vi "Nanotec Controller.vi"(6 "remote":T1) -> ()   [LabVIEW 2023, in "Nanotec Controller.lvlib"]
uses:
  Nanotec Controller.lvlib
  controls/Drive-Mode.ctl
  controls/Go.ctl
  controls/Velocity Pams.ctl
  controls/Units.ctl
  controls/Exps.ctl
  controls/Times.ctl
  controls/Profile Position Units.ctl
  <extravilib>/ChannelInstances/Messenger-t'Message Queue.lvlib-Message Cluster.ctl'/))Channel.ctl
  CMH-Lib/Message Queue/Message Cluster.ctl
  CMH-Lib/Message Queue/Enqueue Multiple Messages.vi
  <extravilib>/ChannelInstances/Messenger-t'Message Queue.lvlib-Message Cluster.ctl'/Read.vi
  <extravilib>/ChannelInstances/Messenger-t'Message Queue.lvlib-Message Cluster.ctl'/Write With Abort.vi
  <extravilib>/ChannelInstances/Messenger-t'Message Queue.lvlib-Message Cluster.ctl'/Read With Abort.vi
  <extravilib>/ChannelInstances/Event Messenger-bool/Instantiate.vi
  <extravilib>/ChannelInstances/Event Messenger-bool/))Channel.vi
  <extravilib>/ChannelInstances/Messenger-t'Message Queue.lvlib-Message Cluster.ctl'/Endpoint.vi
  <vilib>/Utility/error.llb/Error Cluster From Error Code.vi
  <vilib>/ErrorRing/Error Ring.xnode
  CMH-Lib/Message Queue.lvlib
  <extravilib>/ChannelInstances/Event Messenger-bool.lvlib
  NanoLibDLL.dll
  CMH-Lib/Message Queue Helper.lvlib
  <extravilib>/ChannelInstances/Messenger-t'Message Queue.lvlib-Message Cluster.ctl'.lvlib
panel:
  out "Log":string
  out "error out":errorcluster
  in  "Connection Status Control":enum32{"Connection", "Status"}(tab)
  in  "Connect Button":bool
  in  "Ports":i32(listbox)
  in  "Devices":i32(listbox)
  in  "Reboot Device":bool
  out "Connected":bool
  out "NanoJ: STOPPED":bool
  out "Fault":bool
  out "Closed loop available":bool
  out "6041 Bit 13":bool
  out "Warning":bool
  out "Target reached":bool
  out "Internal limit reached":bool
  out "6041 Bit 12":bool
  out "Quick Stop":bool
  out "Voltage enabled":bool
  out "CiA 402 State":string
  out "Mode":string
  in  "Auto-refresh":bool
  out "Current Position":i32
  in  "Get Exceptions":bool
  in  "Get Error Stack":bool
  in  "Device Error Stack":i32(listbox)
  in  "Quick Stop":bool
  in  "Mode Control":T2(tab)
  in  "Open Loop Idle Current (mA)":u32
  in  "Set Motor Settings Button":bool
  in  "Save Motorpams Button":bool
  in  "Auto-Setup Motor Parameters":bool
  in  "Pole Pair Count":u32
  in  "Max Duration (ms)":u32
  in  "Max Current (mA)":u32
  in  "Rated Current (mA)":u32
  in  "Drive-Mode":T3=8 items=["BLDC"=65, "Stepper Closed Loop"=1, "Stepper Open Loop without current-reduction"=0, "Stepper Open Loop with current-reduction"=8]
  in  "Profile Position Units":T4 {"Positioning Exp" items=["10^6"=6, "10^5"=5, "10^4"=4, "10^3"=3, "10^2"=2, "10^1"=1, "10^0"=0, "10^-1"=255, "10^-2"=254, "10^-3"=253, "10^-4"=252, "10^-5"=251, "10^-6"=250]; "Positioning Unit" items=["meter"=1, "inch"=193, "foot"=194, "grade"=64, "radian"=16, "degree"=65, "arcminute"=66, "arcsecond"=67, "mechanical rev"=180]}
  in  "Profile Velocity Units":T8 {"Velocity Time" items=["second"=3, "minute"=71, "hour"=72, "day"=73, "year"=74]; "Velocity Exp" items=["10^6"=6, "10^5"=5, "10^4"=4, "10^3"=3, "10^2"=2, "10^1"=1, "10^0"=0, "10^-1"=255, "10^-2"=254, "10^-3"=253, "10^-4"=252, "10^-5"=251, "10^-6"=250]; "Velocity Unit" items=["meter"=1, "inch"=193, "foot"=194, "grade"=64, "radian"=16, "degree"=65, "arcminute"=66, "arcsecond"=67, "mechanical rev"=180]}
  in  "Gear Ratio Shaft Revs":u32
  in  "Gear Ratio Motor Revs":u32
  in  "Shaft Revolutions":u32
  in  "Save User Units Button":bool
  in  "Set User Units Button":bool
  in  "Feed Constant Per":u32
  in  "Absolute/Relative":u32(ring) items=["Absolute", "Relative"]
  out "Set Position":i32
  in  "Profile Velocity":u32=1
  in  "Halt Positioning Button":bool
  in  "Start Positioning Button":T9
  in  "Target":i32(slide)
  in  "Save Velocity Pams":bool
  in  "Set Velocity Pams":bool
  in  "Velocity Pams":T10={"Target Velocity"=1, "Delta Speed Acc"=1, "Delta Time Acc"=1, "DeltaSpeed Dec"=1, "DeltaTime Dec"=1}
  out "Velocity Demanded":i16
  out "Velocity Actual":i16
  in  "Halt Velocity Button":bool
  in  "Start Velocity Button":T9
  in  "Homing Method":u32(ring)=17 items=["Referencing Negative Switch"=17]
  in  "Speed Switch":u32=3
  in  "Speed Zeroing":u32=2
  in  "Home Button":bool
  in  "Exceptions":i32(listbox)
  in  "Exit":bool
  # "ONLY NECESSARY AFTER\nMOTOR CHANGE"
  # "Position in User Units"
  # "1/min"
  # "<"
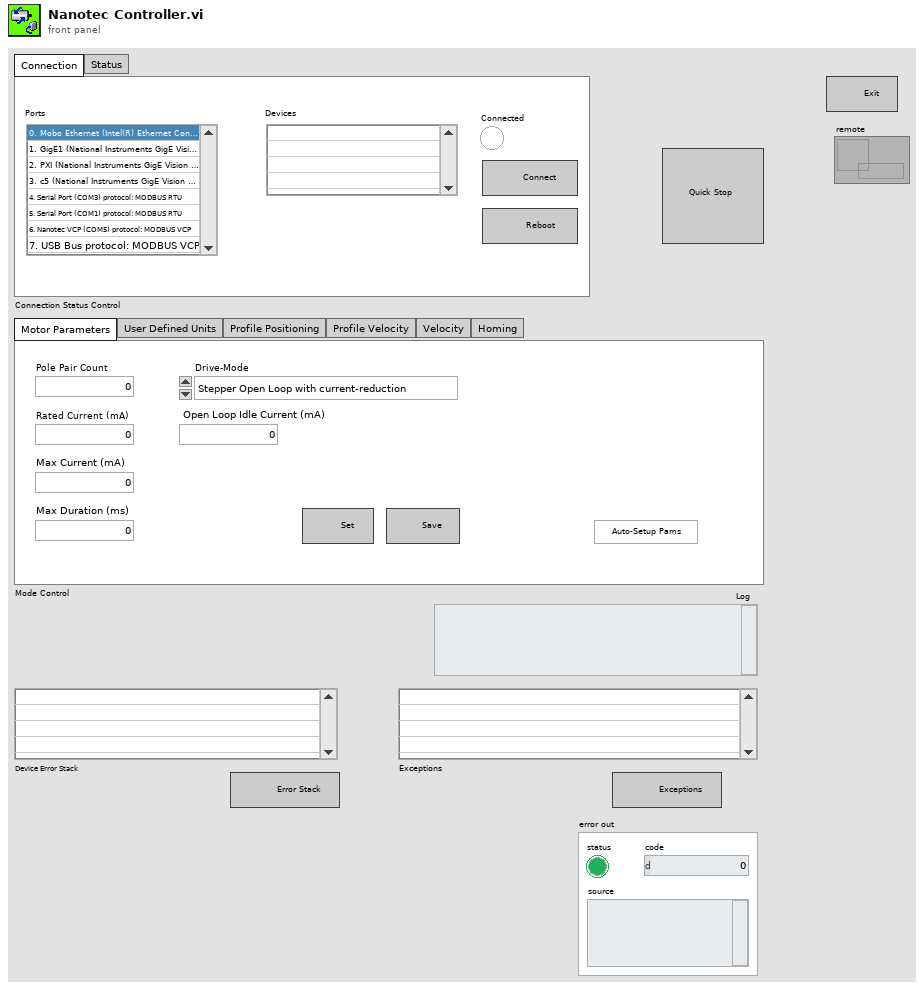
[diagram p1: front panel]
types:
  T1 = typedef "Messenger-t'Message Queue.lvlib-Message Cluster.ctl'.lvlib/))Channel.ctl" = refnum<queue>
  T2 = enum32{"Motor Parameters", "User Defined Units", "Profile Positioning", "Profile Velocity", "Velocity", "Homing"}
  T3 = typedef "Nanotec Controller.lvlib/Drive-Mode.ctl" = u32
  T4 = typedef "Nanotec Controller.lvlib/Profile Position Units.ctl" = cluster{"Positioning Unit":T5, "Positioning Exp":T6}
  T5 = typedef "Nanotec Controller.lvlib/Units.ctl" = u32
  T6 = typedef "Nanotec Controller.lvlib/Exps.ctl" = u32
  T7 = typedef "Nanotec Controller.lvlib/Times.ctl" = u32
  T8 = cluster{"Velocity Unit":T5, "Velocity Exp":T6, "Velocity Time":T7}
  T9 = typedef "Nanotec Controller.lvlib/Go.ctl" = bool
  T10 = typedef "Nanotec Controller.lvlib/Velocity Pams.ctl" = cluster{"Target Velocity":i16, "Delta Speed Acc":u32, "Delta Time Acc":u16, "DeltaSpeed Dec":u32, "DeltaTime Dec":u16}
  T11 = cluster{"Target Velocity":i16, "Delta Speed Acc":u32, "Delta Time Acc":u16, "DeltaSpeed Dec":u32, "DeltaTime Dec":u16}
  T12 = typedef "Event Messenger-bool.lvlib/))Channel.ctl" = refnum<queue>
  T13 = cluster{"velUnit":u32, "velExp":u32, "velTime":u32}
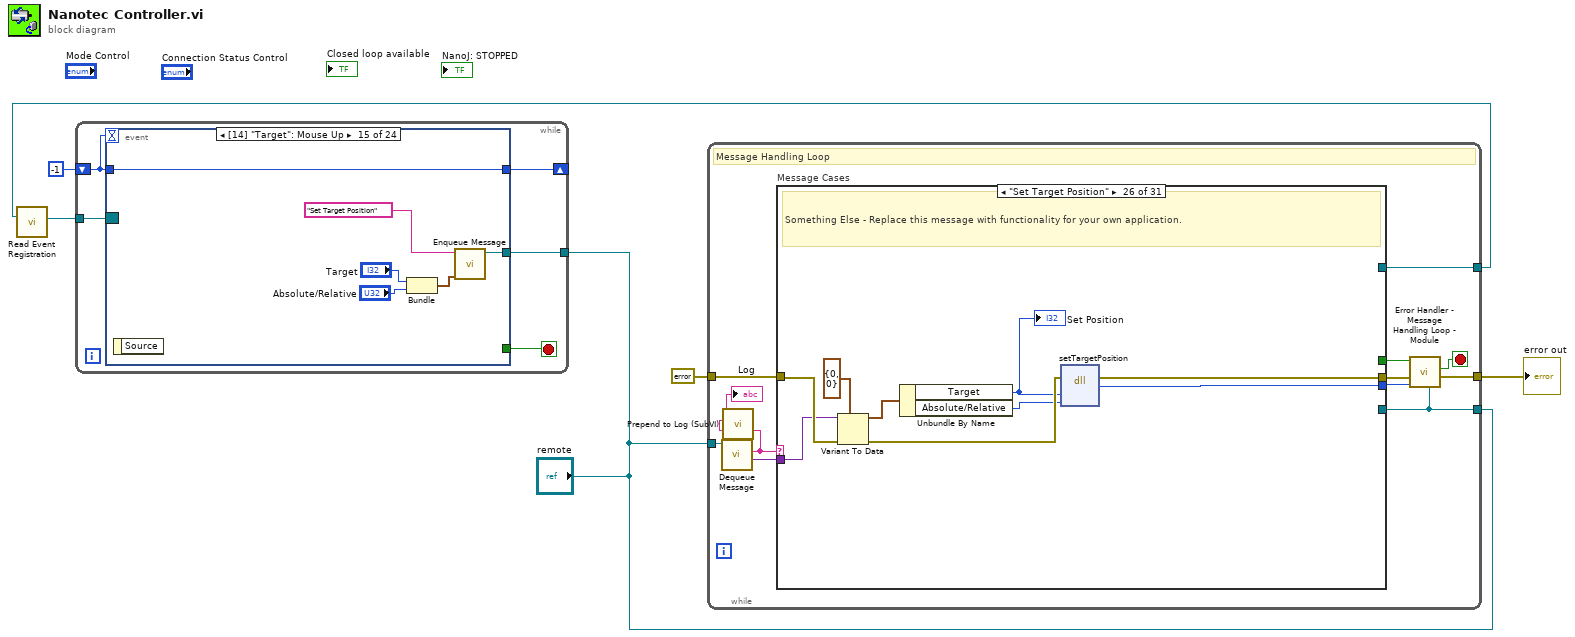
[diagram p0: block diagram]
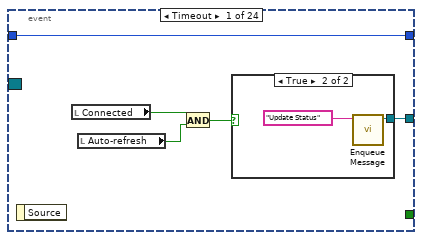
[diagram p2: hidden frame]
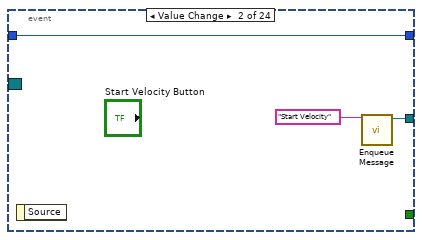
[diagram p4: hidden frame]
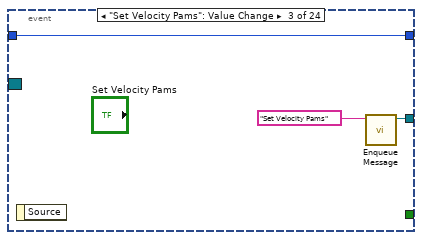
[diagram p5: hidden frame]
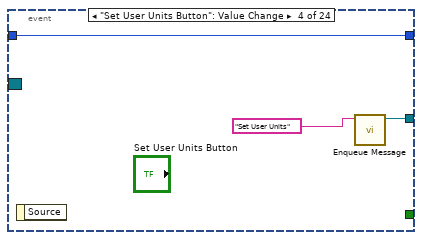
[diagram p6: hidden frame]
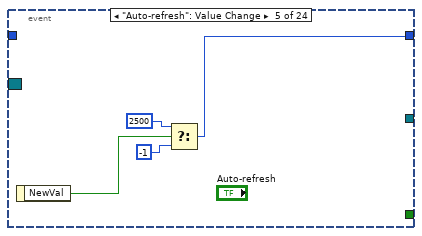
[diagram p7: hidden frame]
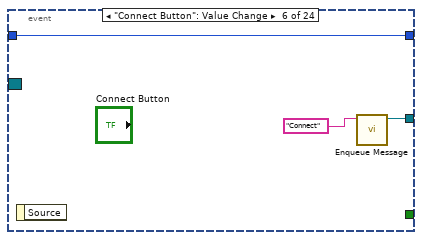
[diagram p8: hidden frame]
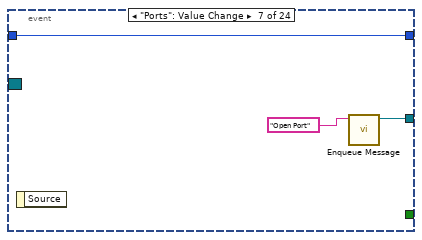
[diagram p9: hidden frame]
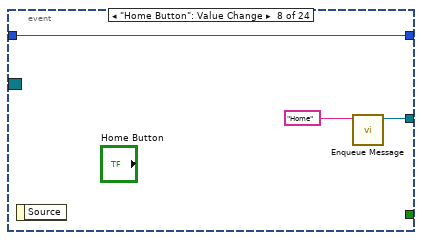
[diagram p10: hidden frame]
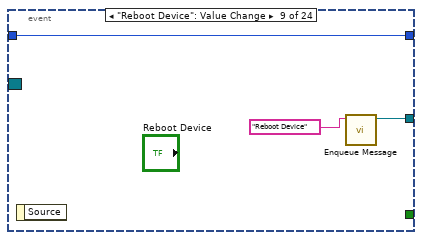
[diagram p11: hidden frame]
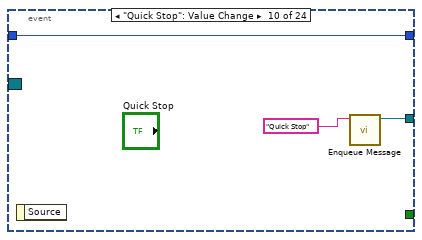
[diagram p12: hidden frame]
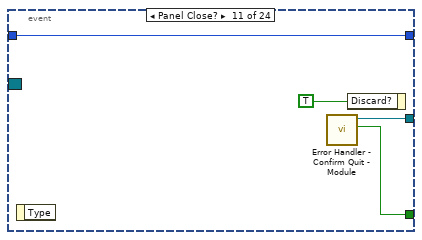
[diagram p13: hidden frame]
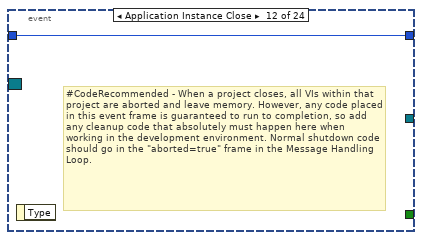
[diagram p14: hidden frame]
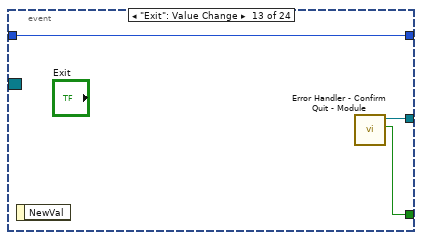
[diagram p15: hidden frame]
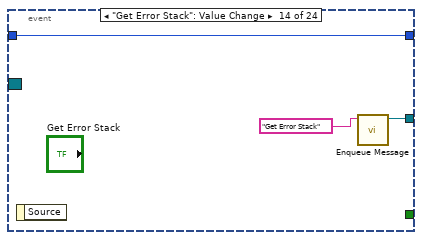
[diagram p16: hidden frame]
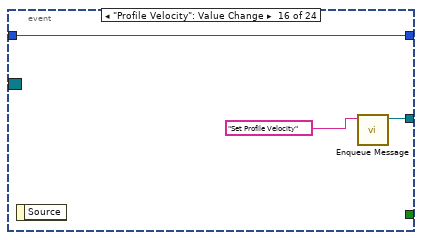
[diagram p17: hidden frame]
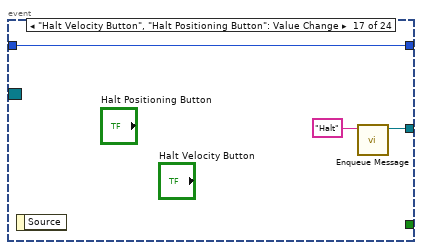
[diagram p18: hidden frame]
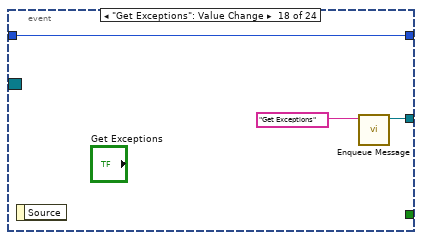
[diagram p19: hidden frame]
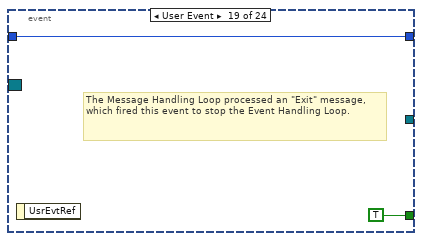
[diagram p20: hidden frame]
diagram:
  n1 = while {
    tunnel: [w15] -> w6
    tunnel: "remote" -> [w17]
    tunnel: errorcluster {"status"=FALSE, "code"=0, "source"=""} ("error IO") -> [w18]
    tunnel: "remote" -> [w7]
    tunnel: [w8] -> w2
    stop <- w12 stop-if-true
    # "Message Handling Loop"
    n2 = call "Dequeue Message.vi"("channel"=w17) -> ("message data"=w16:variant, "message"=w14:string)  [unwired: 8 in, 1 out]
    n3 = call "Prepend to Log (SubVI).vi"("new entry"=w14) -> ("Log out"=→"Log":string)  [unwired: 10 in]
    n4 = case "Message Cases" shown="\"Set Target Position\"" w14 {
      selector: w14 -> [_ _ _ _ _ _ _ _ _ _ _ _ _ _ _ _ _ _ _ _ _ _ _ _ _ _ _ _ _ _ w247]
      tunnel: w18 -> [w19 w27 w37 w46 w49 w55 w71 w74 w84 w91 w100 w105 w108 w129 w132 w136 w141 w153 w157 w161 w167 w170 w174 w189 w193 w200 w216 w219 w222 w243 _]
      tunnel: [w19 w21 w36 w45 w48 w54 w66 w73 w78 w85 w99 w104 w110 w128 w131 w137 w145 w151 w158 w162 w165 w169 w175 w188 w192 w202 w215 w218 w221 w225 w248] -> w10
      tunnel: w16 -> [_ w26 _ _ _ _ w70 _ _ _ _ _ _ _ _ _ _ _ _ _ _ _ _ _ _ w199 _ _ _ _ _]
      tunnel: [_ _ _ _ _ w50 w65 _ _ _ _ _ _ _ _ _ w147 w148 _ _ _ _ _ _ _ _ _ _ _ _ _] -> w7
      tunnel: [_ _ w35 w44 w47 w51 _ w72 _ _ w98 w103 w106 w127 w130 w135 _ w149 w156 w160 w166 w168 w171 w187 w191 w201 w214 w217 w220 w244 _] -> w11
      tunnel: [_ _ _ _ _ _ _ w76 _ _ _ _ _ _ _ _ _ _ _ _ _ _ _ _ _ _ _ _ _ _ _] -> w15
      tunnel: [_ _ _ _ _ _ _ TRUE _ _ _ _ _ _ _ _ FALSE _ _ _ _ _ _ _ _ _ _ _ _ _ _] -> w9
      frame "---Copy This Frame---" {
        # "Duplicate this frame when creating new messages.  Change this comment in the duplicated frame to describe this message."
      }
      frame "Log" {
        # "Duplicate this frame when creating new messages.  Change this comment in the duplicated frame to describe this message."
        n5 = Variant To Data(error in=w27, type="", Variant=w26) -> (data=w22:string, error out=w21:errorcluster)
        n6 = local read "Log"() -> (w24:string)
        n7 = Concatenate Strings(w22, "\r", w24) -> (w20:string)
        n8 = local write "Log"(w20) -> ()
      }
      frame "Get Velocity Pams" {
        # "Duplicate this frame when creating new messages.  Change this comment in the duplicated frame to describe this message."
        n9 = dll-call lib="NanoLibDLL.dll" fn="getVelocityPams"(error in=w37) -> (error out=w36:errorcluster, "success"=w35:i32, "targetVel"=w33:i16, "deltaSpeedAcc"=w32:u32, "deltaTimeAcc"=w31:u16, "deltaSpeedDec"=w30:u32, "deltaTimeDec"=w29:u16)  [unwired: 7 in, 1 out]
        n10 = Bundle By Name(cluster=T11 {"Target Velocity"=1, "Delta Speed Acc"=1, "Delta Time Acc"=1, "DeltaSpeed Dec"=1, "DeltaTime Dec"=1} ("Velocity Pams"), "Target Velocity"=w33, "Delta Speed Acc"=w32, "Delta Time Acc"=w31, "DeltaSpeed Dec"=w30, "DeltaTime Dec"=w29) -> (w28:T11)
        n11 = local write "Velocity Pams"(w28) -> ()
      }
      frame "Set Velocity Pams" {
        # "Duplicate this frame when creating new messages.  Change this comment in the duplicated frame to describe this message."
        n12 = Unbundle By Name("Velocity Pams") -> ("Target Velocity"=w42:i16, "Delta Speed Acc"=w41:u32, "Delta Time Acc"=w40:u16, "DeltaSpeed Dec"=w39:u32, "DeltaTime Dec"=w38:u16)
        n13 = dll-call lib="NanoLibDLL.dll" fn="setVelocityPams"(error in=w46, "targetVel"=w42, "deltaSpeedAcc"=w41, "deltaTimeAcc"=w40, "deltaSpeedDec"=w39, "deltaTimeDec"=w38) -> (error out=w45:errorcluster, "success"=w44:i32)  [unwired: 7 in, 1 out]
      }
      frame "Auto-Setup Motor Pams" {
        # "Sets Motor Parameters. Do This Before connecting new motor. After this do Auto-Setup\non unassemblied motor."
        n14 = dll-call lib="NanoLibDLL.dll" fn="autoSetupMotPams"(error in=w49) -> (error out=w48:errorcluster, "success"=w47:i32)  [unwired: 2 in, 1 out]
      }
      frame "Connect" {
        # "Something Else - Replace this message with functionality for your own application."
        n15 = To Unsigned Long Integer(number="Devices") -> (unsigned 32bit integer=w52:u32)
        n16 = dll-call lib="NanoLibDLL.dll" fn="connectDevice"(error in=w55, "device"=w52) -> (error out=w54:errorcluster, "success"=w51:i32)  [unwired: 3 in, 1 out]
        n17 = case shown="0, Default" w51 {
          tunnel: [w61 _] -> w50
          frame 0, Default {
            n18 = Build Array("Get Motor Pams" ("Message"), "Get User Units" ("Message"), "Get Positioning Pams" ("Message"), "Get Velocity Pams" ("Message")) -> (w57:string[])
            n19 = call-poly "Enqueue Message Poly.vi"("cmd array"=w57) -> ("channel"=w61:T1)  [unwired: 10 in]
            "Connected" <- TRUE ("Connected")
          }
          frame 1 {
            n20 = local write "Connected"(FALSE ("Connected")) -> ()
          }
        }
      }
      frame "Error" {
        # "#CodeRecommended - If you ever change the name of this \"Error\" message, you'll need to update the name in the Check Loop Error.vi as well."
        # "#CodeRecommended - Consider creating a system for logging errors in some way. These errors are for notification purposes only. Handling of specific errors should be performed in the message frames that generated the error."
        # "Error - Display an error dialog. This message is sent by the \"Error Handler\" VIs at the end of other loops in this application."
        n21 = Variant To Data(error in=w71, type=errorcluster {"status"=FALSE, "code"=0, "source"=""} ("error constant"), Variant=w70) -> (data=w68:errorcluster, error out=w67:errorcluster)
        n22 = call <vilib>:"Simple Error Handler.vi"("error in (no error)"=w68) -> ()  [unwired: 4 in, 5 out]
        n23 = Merge Errors(w67) -> (w66:errorcluster)
        n24 = call "Enqueue Message.vi"("Message"="Exit") -> ("channel"=w65:T1)  [unwired: 10 in]
      }
      frame "Shutdown" {
        w77 = TRUE  # Exit
        # "disconnectDevice"
        # "Tell the event loop to stop if it has not done so already."
        # "Bring the hardware into a safe state before exiting"
        n25 = dll-call lib="NanoLibDLL.dll" fn="disconnectDevice"(error in=w74) -> (error out=w73:errorcluster, "success"=w72:i32)  [unwired: 2 in, 1 out]
        n26 = call <extravilib>:"Write.vi"("element"=w77) -> ("channel"=w76:T12)  [unwired: 9 in, 1 out]
      }
      frame "Get Error Stack" {
        # "Gets connected controller's error stack"
        n27 = Initialize Array("", 30 ("dimension size")) -> (w81:string[])
        n28 = dll-call lib="NanoLibDLL.dll" fn="getErrorStackLV"(error in=w84, "Exceptions"=w81) -> (error out=w79:errorcluster, "Exceptions"=w80:string[])  [unwired: 3 in, 1 out]
        n29 = property on="Device Error Stack" class="LstBox (strict)"(error in=w79, "Item Names"=w80) -> (error out=w78:errorcluster)  [unwired: 1 in, 1 out]
      }
      frame "Get Exceptions" {
        # "Something Else - Replace this message with functionality for your own application."
        n30 = Initialize Array("", 30 ("dimension size")) -> (w88:string[])
        n31 = dll-call lib="NanoLibDLL.dll" fn="getExceptionsLV"(error in=w91, "Exceptions"=w88) -> (error out=w86:errorcluster, "Exceptions"=w87:string[])  [unwired: 3 in, 1 out]
        n32 = property on="Exceptions" class="LstBox (strict)"(error in=w86, "Item Names"=w87) -> (error out=w85:errorcluster)  [unwired: 1 in, 1 out]
      }
      frame "Get Motor Pams" {
        n33 = dll-call lib="NanoLibDLL.dll" fn="getMotorParameters"(error in=w100) -> (error out=w99:errorcluster, "success"=w98:i32, "polePairCount"=w97:u32, "ratedCurrent"=w96:u32, "maxCurrent"=w94:u32, "maxCurrentTime"=w95:u32, "openLoopIdleCurrent"=w92:u32, "driveMode"=w93:u32)  [unwired: 8 in, 1 out]
        n34 = local write "Drive-Mode"(w93) -> ()
        n35 = local write "Pole Pair Count"(w97) -> ()
        n36 = local write "Max Duration (ms)"(w95) -> ()
        n37 = local write "Rated Current (mA)"(w96) -> ()
        n38 = local write "Open Loop Idle Current (mA)"(w92) -> ()
        n39 = local write "Max Current (mA)"(w94) -> ()
      }
      frame "Get Positioning Pams" {
        n40 = dll-call lib="NanoLibDLL.dll" fn="getPositioningParameters"(error in=w105) -> (error out=w104:errorcluster, "success"=w103:i32, "profileVelocity"=w102:u32, "target position"=w101:i32)  [unwired: 4 in, 1 out]
        n41 = local write "Profile Velocity"(w102) -> ()
        n42 = local write "Set Position"(w101) -> ()
      }
      frame "Get Ports" {
        # "Something - Replace this message with functionality for your own application."
        n43 = property on="Ports" class="LstBox (strict)"(error in=w108, "Value"=-1 ("Ports")) -> (error out=w109:errorcluster)  [unwired: 1 in, 1 out]
        n44 = Initialize Array("", 30 ("dimension size")) -> (w112:string[])
        n45 = dll-call lib="NanoLibDLL.dll" fn="getPortsLV"(error in=w109, "ports"=w112) -> (error out=w111:errorcluster, "success"=w106:i32, "ports"=w115:string[])  [unwired: 2 in, 1 out]
        n46 = property on="Ports" class="LstBox (strict)"(error in=w111, "Item Names"=w115) -> (error out=w110:errorcluster)  [unwired: 1 in, 1 out]
      }
      frame "Get User Units" {
        n47 = dll-call lib="NanoLibDLL.dll" fn="getUserUnits"(error in=w129) -> (error out=w128:errorcluster, "success"=w127:i32, "feed"=w126:u32, "shaftRevs"=w125:u32, "posUnit"=w122:u32, "posExp"=w121:u32, "velUnit"=w119:u32, "velExp"=w118:u32, "velTime"=w117:u32, "gearRatioMotorRevs"=w124:u32, "gearRatioShaftRevs"=w123:u32)  [unwired: 11 in, 1 out]
        n48 = local write "Feed Constant Per"(w126) -> ()
        n49 = local write "Shaft Revolutions"(w125) -> ()
        n50 = local write "Gear Ratio Motor Revs"(w124) -> ()
        n51 = local write "Gear Ratio Shaft Revs"(w123) -> ()
        n52 = Bundle("velUnit"=w119, "velExp"=w118, "velTime"=w117) -> (w116:T13)  [unwired: 1 in]
        n53 = Bundle("posUnit"=w122, "posExp"=w121) -> (w120:cluster{"posUnit":u32, "posExp":u32})  [unwired: 1 in]
        n54 = local write "Profile Velocity Units"(w116) -> ()
        n55 = local write "Profile Position Units"(w120) -> ()
      }
      frame "Halt" {
        # "Something Else - Replace this message with functionality for your own application."
        n56 = dll-call lib="NanoLibDLL.dll" fn="halt"(error in=w132) -> (error out=w131:errorcluster, "success"=w130:i32)  [unwired: 2 in, 1 out]
      }
      frame "Home" {
        # "Something - Replace this message with functionality for your own application."
        n57 = dll-call lib="NanoLibDLL.dll" fn="home"(error in=w136, "speedZero"="Speed Zeroing", "speedSwitch"="Speed Switch") -> (error out=w137:errorcluster, "success"=w135:i32)  [unwired: 4 in, 1 out]
      }
      frame "Init" {
        w143 = ""
        w142 = string[] []
        w146 = -1 ("Ports")
        # "Initialize - All initialization work should take place in this message, since other loops can potentially enqueue messages that execute immediately after this one."
        n58 = local write "Mode"(w143) -> ()
        n59 = local write "CiA 402 State"(w143) -> ()
        n60 = local write "Connected"(FALSE ("Connected")) -> ()
        n61 = local write "Auto-refresh"(FALSE ("Auto-refresh")) -> ()
        n62 = property on="Ports" class="LstBox (strict)"("Item Names"=w142) -> ()  [unwired: 2 in, 2 out]
        n63 = property on="Device Error Stack" class="LstBox (strict)"(error in=w141, "Item Names"=w142) -> (error out=w145:errorcluster)  [unwired: 1 in, 1 out]
        n64 = property on="Devices" class="LstBox (strict)"("Item Names"=w142) -> ()  [unwired: 2 in, 2 out]
        n65 = property on="Exceptions" class="LstBox (strict)"("Item Names"=w142) -> ()  [unwired: 2 in, 2 out]
        n66 = local write "Devices"(w146) -> ()
        n67 = local write "Ports"(w146) -> ()
        n68 = call "Enqueue Message.vi"("Message"="Get Ports") -> ("channel"=w147:T1)  [unwired: 10 in]
      }
      frame "Open Port" {
        # "Something Else - Replace this message with functionality for your own application."
        n69 = To Unsigned Long Integer(number="Ports") -> (unsigned 32bit integer=w152:u32)
        n70 = dll-call lib="NanoLibDLL.dll" fn="openPort"(error in=w153, "portToOpen"=w152) -> (error out=w151:errorcluster, "success"=w149:i32)  [unwired: 3 in, 1 out]
        n71 = case shown="0, Default" w149 {
          tunnel: [w155 _] -> w148
          frame 0, Default {
            n72 = call "Enqueue Message.vi"("Message"="Scan Bus") -> ("channel"=w155:T1)  [unwired: 10 in]
          }
          frame 1 {
          }
        }
      }
      frame "Quick Stop" {
        # "Quick Stop uses"
        n73 = dll-call lib="NanoLibDLL.dll" fn="quickStop"(error in=w157) -> (error out=w158:errorcluster, "success"=w156:i32)  [unwired: 2 in, 1 out]
      }
      frame "Reboot Device" {
        # "Something - Replace this message with functionality for your own application."
        n74 = dll-call lib="NanoLibDLL.dll" fn="rebootDevice"(error in=w161) -> (error out=w162:errorcluster, "success"=w160:i32)  [unwired: 2 in, 1 out]
        n75 = case shown="0, Default" w160 {
          tunnel: [FALSE TRUE] -> w159
          frame 0, Default {
          }
          frame 1 {
          }
        }
        n76 = local write "Connected"(w159) -> ()
      }
      frame "Save Motor Pams" {
        # "Bring the hardware into a safe state before exiting"
        n77 = dll-call lib="NanoLibDLL.dll" fn="saveMotorParameters"(error in=w167) -> (error out=w165:errorcluster, "success"=w166:i32)  [unwired: 2 in, 1 out]
      }
      frame "Save User Units" {
        # "Duplicate this frame when creating new messages.  Change this comment in the duplicated frame to describe this message."
        n78 = dll-call lib="NanoLibDLL.dll" fn="saveUserUnits"(error in=w170) -> (error out=w169:errorcluster, "success"=w168:i32)  [unwired: 2 in, 1 out]
      }
      frame "Scan Bus" {
        # "Something - Replace this message with functionality for your own application."
        n79 = property on="Devices" class="LstBox (strict)"(error in=w174, "Value"=-1 ("Devices")) -> (error out=w173:errorcluster)  [unwired: 1 in, 1 out]
        n80 = Initialize Array("", 30 ("dimension size")) -> (w177:string[])
        n81 = dll-call lib="NanoLibDLL.dll" fn="scanBusLV"(error in=w173, "devices"=w177) -> (error out=w176:errorcluster, "success"=w171:i32, "devices"=w180:string[])  [unwired: 2 in, 1 out]
        n82 = property on="Devices" class="LstBox (strict)"(error in=w176, "Item Names"=w180) -> (error out=w175:errorcluster)  [unwired: 1 in, 1 out]
      }
      frame "Set Motor Pams" {
        # "Sets Motor Parameters. Do This Before connecting new motor. After this do Auto-Setup\non unassemblied motor."
        n83 = dll-call lib="NanoLibDLL.dll" fn="setMotorParameters"(error in=w189, "polePairCount"="Pole Pair Count", "ratedCurrent (mA)"="Rated Current (mA)", "maxCurrent (mA)"="Max Current (mA)", "maxCurrentDuration (mA)"="Max Duration (ms)", "openLoopIdleCurrent"="Open Loop Idle Current (mA)", "driveMode"="Drive-Mode") -> (error out=w188:errorcluster, "success"=w187:i32)  [unwired: 8 in, 1 out]
      }
      frame "Set Profile Velocity" {
        # "Something Else - Replace this message with functionality for your own application."
        n84 = dll-call lib="NanoLibDLL.dll" fn="setProfileVelocity"(error in=w193, "profileVelocity"="Profile Velocity") -> (error out=w192:errorcluster, "success"=w191:i32)  [unwired: 3 in, 1 out]
      }
      frame "Set Target Position" {
        # "Something Else - Replace this message with functionality for your own application."
        n85 = Variant To Data(error in=w200, type=cluster{"Target":i32, "Absolute/Relative":u32} {"Target"=0, "Absolute/Relative"=0} ("output cluster"), Variant=w199) -> (data=w197:cluster{"Target":i32, "Absolute/Relative":u32}, error out=w196:errorcluster)
        n86 = Unbundle By Name(w197) -> ("Target"=w194:i32, "Absolute/Relative"=w195:u32)
        "Set Position" <- w194
        n87 = dll-call lib="NanoLibDLL.dll" fn="setTargetPosition"(error in=w196, "position"=w194, "abs/rel"=w195) -> (error out=w202:errorcluster, "success"=w201:i32)  [unwired: 4 in, 1 out]
      }
      frame "Set User Units" {
        n88 = Unbundle("Profile Position Units") -> ("Positioning Unit"=w208:T5, "Positioning Exp"=w207:T6)
        n89 = Unbundle("Profile Velocity Units") -> ("Velocity Unit"=w205:T5, "Velocity Exp"=w204:T6, "Velocity Time"=w203:T7)
        n90 = dll-call lib="NanoLibDLL.dll" fn="setUserUnits"(error in=w216, "feed"="Feed Constant Per", "shaftRevs"="Shaft Revolutions", "posUnit"=w208, "posExp"=w207, "velUnit"=w205, "velExp"=w204, "velTime"=w203, "gearRatioMotorRevs"="Gear Ratio Motor Revs", "gearRatioShaftRevs"="Gear Ratio Shaft Revs") -> (error out=w215:errorcluster, "success"=w214:i32)  [unwired: 11 in, 1 out]
      }
      frame "Start Positioning" {
        # "Something Else - Replace this message with functionality for your own application."
        n91 = dll-call lib="NanoLibDLL.dll" fn="startPositioning"(error in=w219) -> (error out=w218:errorcluster, "success"=w217:i32)  [unwired: 2 in, 1 out]
      }
      frame "Start Velocity" {
        # "Something Else - Replace this message with functionality for your own application."
        n92 = dll-call lib="NanoLibDLL.dll" fn="startVelocity"(error in=w222) -> (error out=w221:errorcluster, "success"=w220:i32)  [unwired: 2 in, 1 out]
      }
      frame "Update Status" {
        # "Read Stati from Controller"
        n93 = dll-call lib="NanoLibDLL.dll" fn="getCiA402StateLV"(error in=w243) -> (error out=w232:errorcluster, "success"=w242:i32, "state"=→"CiA 402 State":string, "Fault"=→"Fault":bool, "Voltage enabled"=→"Voltage enabled":bool, "Quick Stop"=→"Quick Stop":bool, "Warning"=→"Warning":bool, "Target reached"=→"Target reached":bool, "Internal limit reached"=→"Internal limit reached":bool, "6041 Bit 12"=→"6041 Bit 12":bool, "6041 Bit 13"=→"6041 Bit 13":bool)  [unwired: 11 in, 1 out]
        n94 = dll-call lib="NanoLibDLL.dll" fn="getModeOfOperationLV"(error in=w232) -> (error out=w231:errorcluster, "success"=w229:i32, "mode"=→"Mode":string)  [unwired: 3 in, 1 out]
        n95 = dll-call lib="NanoLibDLL.dll" fn="getPositionActual"(error in=w231) -> (error out=w227:errorcluster, "success"=w228:i32, "positionActual"=→"Current Position":i32)  [unwired: 3 in, 1 out]
        n96 = Equal To 0?(x=w242) -> (x = 0?=w241:bool)
        n97 = local write "Connected"(w241) -> ()
        n98 = dll-call lib="NanoLibDLL.dll" fn="getVelocityStatus"(error in=w227) -> (error out=w225:errorcluster, "success"=w226:i32, "velDemanded"=→"Velocity Demanded":i16, "velActual"=→"Velocity Actual":i16)  [unwired: 4 in, 1 out]
        n99 = Compound Arithmetic op=OR(w226, w229, w228, w242) -> (w244:i32)
      }
      frame Default {
        # "'Default' case only runs if there is a message that isn't defined in any of the other cases.  Output a programming error."
        n100 = xnode "Error Ring"("parameter 0"=w247) -> ("error out"=w248:errorcluster)
      }
    }
    n101 = call "Error Handler - Message Handling Loop - Module.vi"("channel"=w7, "DLL success"=w11, "error in (no error)"=w10, "Shutdown?"=w9) -> ("dup error in"=w8:errorcluster, "Shutdown!"=w12:bool)  [unwired: 6 in]
  }
  "error out" <- w2
  n102 = call <extravilib>:"Read Event Registration.vi"("channel"=w6) -> ("event registration refnum"=w4:refnum<event-registration>)  [unwired: 10 in]
  n103 = while {
    tunnel: w4 -> [w260]
    tunnel: "remote" -> [w259]
    shift-right: [w257] -> _
    shift-left: -1 -> [w256]
    stop <- w258 stop-if-true
    n104 = event shown="[14] \"Target\": Mouse Up" {
      selector: w260 -> [_ _ _ _ _ _ _ _ _ _ _ _ _ _ _ _ _ _ _ _ _ _ _ _]
      dyn-events: _ -> [_ _ _ _ _ _ _ _ _ _ _ _ _ _ _ _ _ _ _ _ _ _ _ _]
      timeout: w256 -> [_ _ _ _ _ _ _ _ _ _ _ _ _ _ _ _ _ _ _ _ _ _ _ _]
      tunnel: [_ _ _ _ _ _ _ _ _ _ w297 _ w302 _ _ _ _ _ TRUE ("Discard?") _ _ _ _ _] -> w258
      tunnel: [w265 w269 w271 w276 _ w283 w286 w289 w292 w295 w298 _ w303 w306 w312 w315 w318 w321 _ w326 w329 w332 w337 w340] -> w259
      tunnel: [w263 w268 w272 w275 w277 w282 w285 w288 w291 w294 w296 w300 w301 w305 w311 w314 w317 w320 w322 w325 w328 w333 w336 w339] -> w257
      tunnel: w256 -> [w263 w268 w272 w275 _ w282 w285 w288 w291 w294 w296 w300 w301 w305 w311 w314 w317 w320 w322 w325 w328 w333 w336 w339]
      event Timeout {
        n105 = event-data() -> ()  [unwired: 1 in, 1 out]
        n106 = local read "Connected"() -> (w264:bool)
        n107 = local read "Auto-refresh"() -> (w261:bool)
        n108 = And(x=w264, y=w261) -> (x .and. y?=w262:bool)
        n109 = case shown="True" w262 {
          tunnel: [_ w267] -> w265
          frame False {
          }
          frame True {
            n110 = call "Enqueue Message.vi"("Message"="Update Status") -> ("channel"=w267:T1)  [unwired: 10 in]
          }
        }
      }
      event Value Change {
        n111 = event-data() -> ()  [unwired: 1 in, 1 out]
        n112 = call "Enqueue Message.vi"("Message"="Start Velocity") -> ("channel"=w269:T1)  [unwired: 10 in]
      }
      event "Set Velocity Pams": Value Change {
        n113 = event-data() -> ()  [unwired: 1 in, 1 out]
        n114 = call "Enqueue Message.vi"("Message"="Set Velocity Pams") -> ("channel"=w271:T1)  [unwired: 10 in]
      }
      event "Set User Units Button": Value Change {
        n115 = event-data() -> ()  [unwired: 1 in, 1 out]
        n116 = call "Enqueue Message.vi"("Message"="Set User Units") -> ("channel"=w276:T1)  [unwired: 10 in]
      }
      event "Auto-refresh": Value Change {
        n117 = event-data() -> ("NewVal"=w280:bool)  [unwired: 1 in]
        n118 = Select(t=2500, s=w280, f=-1) -> (s? t:f=w277:i32)
      }
      event "Connect Button": Value Change {
        n119 = event-data() -> ()  [unwired: 1 in, 1 out]
        n120 = call "Enqueue Message.vi"("Message"="Connect") -> ("channel"=w283:T1)  [unwired: 10 in]
      }
      event "Ports": Value Change {
        n121 = event-data() -> ()  [unwired: 1 in, 1 out]
        n122 = call "Enqueue Message.vi"("Message"="Open Port") -> ("channel"=w286:T1)  [unwired: 10 in]
      }
      event "Home Button": Value Change {
        n123 = event-data() -> ()  [unwired: 1 in, 1 out]
        n124 = call "Enqueue Message.vi"("Message"="Home") -> ("channel"=w289:T1)  [unwired: 10 in]
      }
      event "Reboot Device": Value Change {
        n125 = event-data() -> ()  [unwired: 1 in, 1 out]
        n126 = call "Enqueue Message.vi"("Message"="Reboot Device") -> ("channel"=w292:T1)  [unwired: 10 in]
      }
      event "Quick Stop": Value Change {
        n127 = event-data() -> ()  [unwired: 1 in, 1 out]
        n128 = call "Enqueue Message.vi"("Message"="Quick Stop") -> ("channel"=w295:T1)  [unwired: 10 in]
      }
      event Panel Close? {
        n129 = event-data() -> ()  [unwired: 1 in, 1 out]
        n130 = call "Error Handler - Confirm Quit - Module.vi"() -> ("exit confirmed"=w297:bool, "channel"=w298:T1)  [unwired: 10 in]
        n131 = event-data("Discard?"=TRUE) -> ()  [unwired: 1 in, 1 out]
      }
      event Application Instance Close {
        # "#CodeRecommended - When a project closes, all VIs within that project are aborted and leave memory. However, any code placed in this event frame is guaranteed to run to completion, so add any cleanup code that absolutely must happen here when working in the development environment. Normal shutdown code should go in the \"aborted=true\" frame in the Message Handling Loop."
        n132 = event-data() -> ()  [unwired: 1 in, 1 out]
      }
      event "Exit": Value Change {
        n133 = event-data() -> ()  [unwired: 1 in, 1 out]
        n134 = call "Error Handler - Confirm Quit - Module.vi"() -> ("exit confirmed"=w302:bool, "channel"=w303:T1)  [unwired: 10 in]
      }
      event "Get Error Stack": Value Change {
        n135 = event-data() -> ()  [unwired: 1 in, 1 out]
        n136 = call "Enqueue Message.vi"("Message"="Get Error Stack") -> ("channel"=w306:T1)  [unwired: 10 in]
      }
      event "Target": Mouse Up {
        n137 = event-data() -> ()  [unwired: 1 in, 1 out]
        n138 = Bundle("Target"="Target", "Absolute/Relative"="Absolute/Relative") -> (w307:cluster{"Target":i32, "Absolute/Relative":u32})  [unwired: 1 in]
        n139 = call "Enqueue Message.vi"("Message Data"=w307, "Message"="Set Target Position") -> ("channel"=w312:T1)  [unwired: 9 in]
      }
      event "Profile Velocity": Value Change {
        n140 = event-data() -> ()  [unwired: 1 in, 1 out]
        n141 = call "Enqueue Message.vi"("Message"="Set Profile Velocity") -> ("channel"=w315:T1)  [unwired: 10 in]
      }
      event "Halt Velocity Button", "Halt Positioning Button": Value Change {
        n142 = event-data() -> ()  [unwired: 1 in, 1 out]
        n143 = call "Enqueue Message.vi"("Message"="Halt") -> ("channel"=w318:T1)  [unwired: 10 in]
      }
      event "Get Exceptions": Value Change {
        n144 = event-data() -> ()  [unwired: 1 in, 1 out]
        n145 = call "Enqueue Message.vi"("Message"="Get Exceptions") -> ("channel"=w321:T1)  [unwired: 10 in]
      }
      event User Event {
        # "The Message Handling Loop processed an \"Exit\" message, which fired this event to stop the Event Handling Loop."
        n146 = event-data() -> ()  [unwired: 1 in, 1 out]
      }
      event "Set Motor Settings Button": Value Change {
        n147 = event-data() -> ()  [unwired: 1 in, 1 out]
        n148 = call "Enqueue Message.vi"("Message"="Set Motor Pams") -> ("channel"=w326:T1)  [unwired: 10 in]
      }
      event Value Change {
        n149 = event-data() -> ()  [unwired: 1 in, 1 out]
        n150 = call "Enqueue Message.vi"("Message"="Start Positioning") -> ("channel"=w329:T1)  [unwired: 10 in]
      }
      event "Save Motorpams Button": Value Change {
        n151 = event-data() -> ()  [unwired: 1 in, 1 out]
        n152 = Build Array("Save Motor Pams" ("Message"), "Save User Units" ("Message")) -> (w330:string[])
        n153 = call-poly "Enqueue Message Poly.vi"("cmd array"=w330) -> ("channel"=w332:T1)  [unwired: 10 in]
      }
      event "Save User Units Button", "Save Velocity Pams": Value Change {
        n154 = event-data() -> ()  [unwired: 1 in, 1 out]
        n155 = call "Enqueue Message.vi"("Message"="Save User Units") -> ("channel"=w337:T1)  [unwired: 10 in]
      }
      event "Auto-Setup Motor Parameters": Value Change {
        n156 = event-data() -> ()  [unwired: 1 in, 1 out]
        n157 = call "Enqueue Message.vi"("Message"="Auto-Setup Motor Pams") -> ("channel"=w340:T1)  [unwired: 10 in]
      }
    }
  }
